vi "On-board IO.vi"(10 "O/P":T1) -> (2 "I/P":T2 {"X-Axis" scale=-15.0..15.0; "Y-Axis" scale=-15.0..15.0; "Z-Axis" scale=-15.0..15.0})   [LabVIEW 2015]
uses:
  <vilib>/eio/EIONode/EIONode.xnode
  <vilib>/rvi/eio/common/nirviEmuTemplateMethod_errors.vi
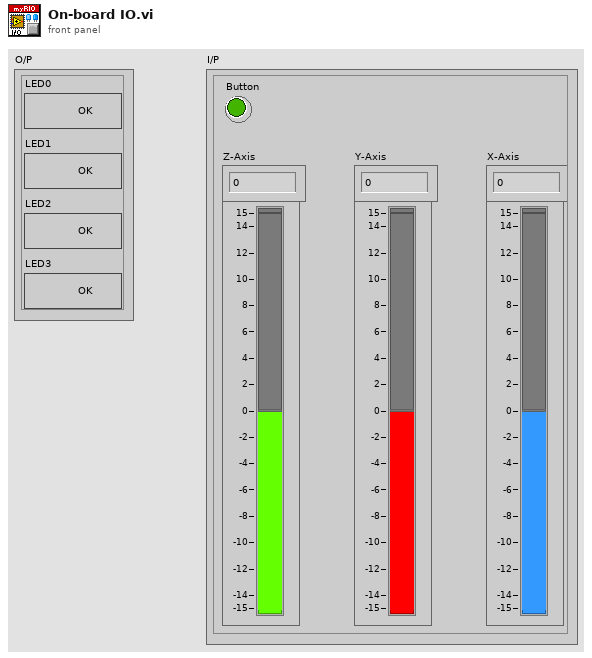
[diagram p1: front panel]
types:
  T1 = cluster{"LED0":bool, "LED1":bool, "LED2":bool, "LED3":bool}
  T2 = cluster{"Button":bool, "Z-Axis":i16, "Y-Axis":i16, "X-Axis":i16}
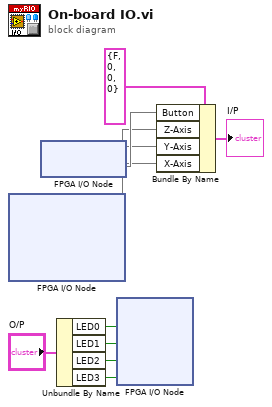
[diagram p0: block diagram]
diagram:
  n1 = xnode "FPGA I/O Node"() -> ("AccelerationX"=w7, "AccelerationY"=w8, "AccelerationZ"=w9)  [unwired: 4 in, 5 out]
  n2 = xnode "FPGA I/O Node"() -> ("Button0"=w10)  [unwired: 1 in, 1 out]
  n3 = Unbundle By Name("O/P") -> ("LED0"=w4:bool, "LED1"=w3:bool, "LED2"=w2:bool, "LED3"=w1:bool)
  n4 = xnode "FPGA I/O Node"("LED0"=w4, "LED1"=w3, "LED2"=w2, "LED3"=w1) -> ()  [unwired: 4 in, 4 out]
  n5 = Bundle By Name(cluster=T2 {"Button"=FALSE, "Z-Axis"=0, "Y-Axis"=0, "X-Axis"=0} ("O/P"), "Button"=w10, "Z-Axis"=w9, "Y-Axis"=w8, "X-Axis"=w7) -> (→"I/P":T2)
